vi "toml_to_value.vi"(8 "error in (no error)":errorcluster, 11 "toml line":string) -> (0 "error out":errorcluster, 1 "remaining":string, 2 "arg":string, 3 "token":T1)   [LabVIEW 2017]
uses:
  toml_token.ctl
  <vilib>/regexp/Match Regular Expression.xnode
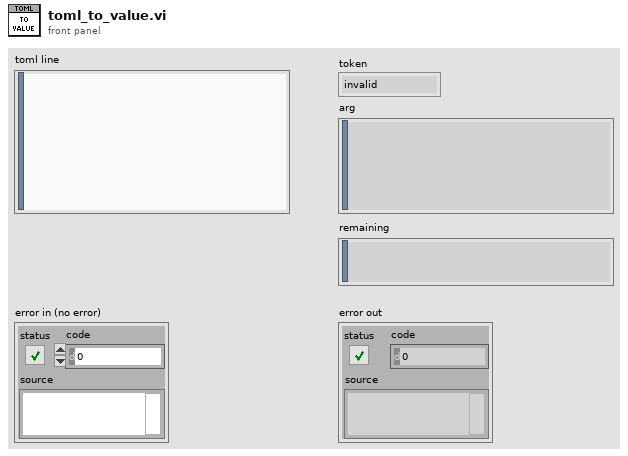
[diagram p1: front panel]
types:
  T1 = typedef "toml_token.ctl" = enum8{"invalid", "bool", "string", "string_start", "int", "uint", "float", "datetime", "array", "inline_table", "table", "table_element", "key", "comment", "comment_inline", "end"}
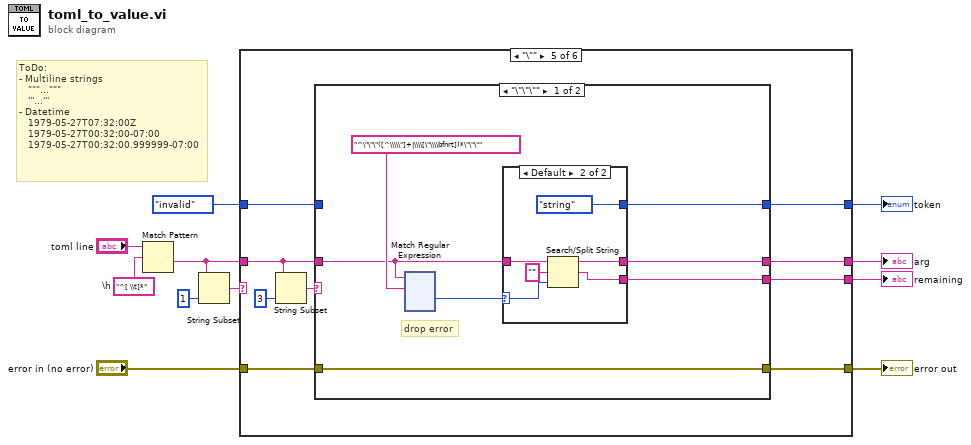
[diagram p0: block diagram]
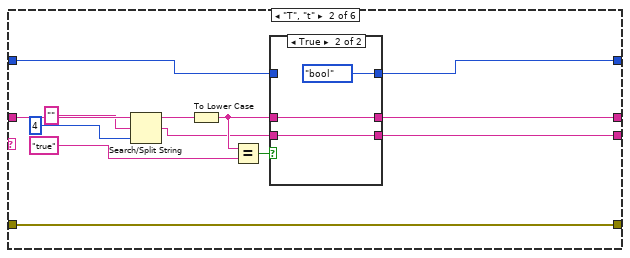
[diagram p3: hidden frame]
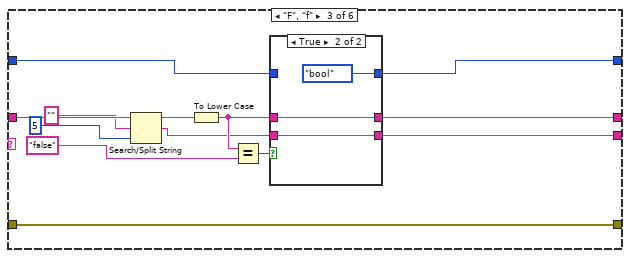
[diagram p5: hidden frame]
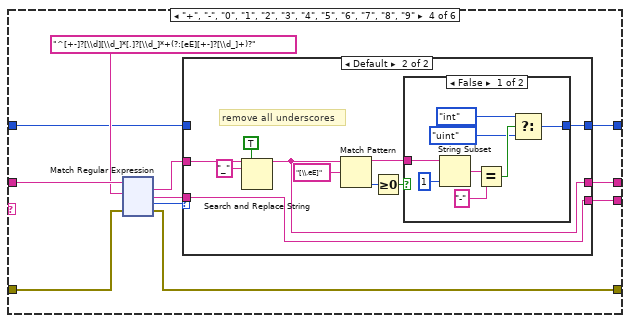
[diagram p7: hidden frame]
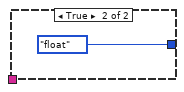
[diagram p9: hidden frame]
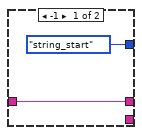
[diagram p10: hidden frame]
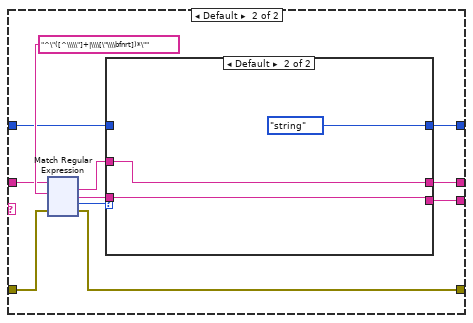
[diagram p11: hidden frame]
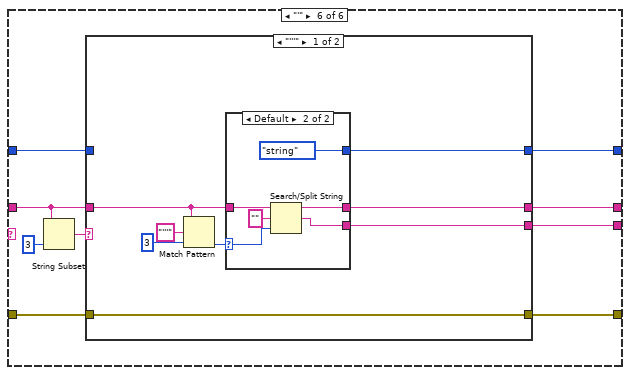
[diagram p13: hidden frame]
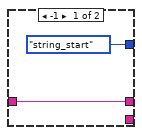
[diagram p14: hidden frame]
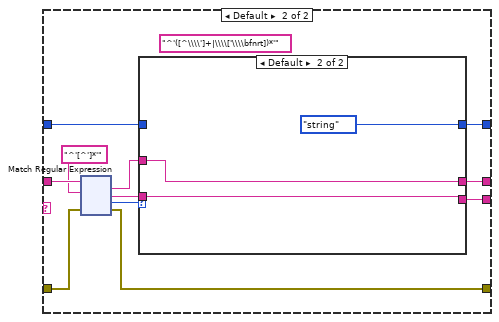
[diagram p15: hidden frame]
diagram:
  w11 = "^[ \\t]*"  # \h
  # "ToDo:\n- Multiline strings \n   \"\"\"...\"\"\"\n   '''...'''\n- Datetime\n   1979-05-27T07:32:00Z\n   1979-05-27T00:32:00-07:00\n   1979-05-27T00:32:00.999999-07:00"
  n1 = Match Pattern(string="toml line", regular expression=w11) -> (after substring=w7:string)  [unwired: 1 in, 3 out]
  n2 = String Subset(string=w7, length (rest)=1 ("length (rest)")) -> (substring=w8:string)  [unwired: 1 in]
  n3 = case shown="\"\\\"\"" w8 {
    tunnel: w7 -> [_ w25 w42 w58 w194 w461]
    tunnel: [_ w18 w35 w50 w197 w464] -> w6
    tunnel: [_ w15 w32 w49 w196 w463] -> w5
    tunnel: [w13 w21 w38 w53 w199 w466] -> w4
    tunnel: toml_token."invalid" ("token") -> [w13 w14 w31 w52 w198 w465]
    tunnel: [w12 w20 w37 w55 w200 w467] -> w2
    tunnel: "error in (no error)" -> [w12 w20 w37 w56 w201 w468]
    frame Default {
    }
    frame "T", "t" {
      n4 = Search/Split String(string=w25, search string/char (-)="", offset (0)=4 ("length (rest)")) -> (substring before match=w22:string, match + rest of string=w16:string)  [unwired: 1 out]
      n5 = To Lower Case(string=w22) -> (all lower case string=w17:string)
      n6 = Equal?(x=w17, y="true") -> (x = y?=w19:bool)
      n7 = case shown="True" w19 {
        tunnel: [w27 toml_token."bool" ("token")] -> w21
        tunnel: [_ w29] -> w18
        tunnel: w17 -> [_ w29]
        tunnel: w16 -> [_ w28]
        tunnel: [_ w28] -> w15
        tunnel: w14 -> [w27 _]
        frame False {
        }
        frame True {
        }
      }
    }
    frame "F", "f" {
      n8 = Search/Split String(string=w42, search string/char (-)="", offset (0)=5 ("length (rest)")) -> (substring before match=w39:string, match + rest of string=w33:string)  [unwired: 1 out]
      n9 = To Lower Case(string=w39) -> (all lower case string=w34:string)
      n10 = Equal?(x=w34, y="false") -> (x = y?=w36:bool)
      n11 = case shown="True" w36 {
        tunnel: [w44 toml_token."bool" ("token")] -> w38
        tunnel: [_ w46] -> w35
        tunnel: w34 -> [_ w46]
        tunnel: w33 -> [_ w45]
        tunnel: [_ w45] -> w32
        tunnel: w31 -> [w44 _]
        frame False {
        }
        frame True {
        }
      }
    }
    frame "+", "-", "0", "1", "2", "3", "4", "5", "6", "7", "8", "9" {
      n12 = xnode "Match Regular Expression"("input string"=w58, "regular expression"="^[+-]?[\\d][\\d_]*[.]?[\\d_]*+(?:[eE][+-]?[\\d_]+)?", "error in"=w56) -> ("whole match"=w51:string, "after match"=w48:string, "offset past match"=w54:i32, "error out"=w55:errorcluster)  [unwired: 3 in, 1 out]
      n13 = case shown="Default" w54 {
        tunnel: [w59 w65] -> w53
        tunnel: w52 -> [w59 _]
        tunnel: w51 -> [_ w63]
        tunnel: [_ w62] -> w50
        tunnel: [_ w64] -> w49
        tunnel: w48 -> [_ w64]
        frame -1 {
        }
        frame Default {
          # "remove all underscores"
          n14 = Search and Replace String(replace all?=TRUE ("replace all? (F)"), input string=w63, search string="_") -> (result string=w62:string)  [unwired: 5 in, 3 out]
          n15 = Match Pattern(string=w62, regular expression="[\\.eE]") -> (before substring=w66:string, offset past match=w68:i32)  [unwired: 1 in, 2 out]
          n16 = Greater Or Equal To 0?(x=w68) -> (x >= 0?=w67:bool)
          n17 = case shown="False" w67 {
            tunnel: w66 -> [w77 _]
            tunnel: [w72 toml_token."float" ("token")] -> w65
            frame False {
              n18 = String Subset(string=w77, length (rest)=1 ("length (rest)")) -> (substring=w75:string)  [unwired: 1 in]
              n19 = Equal?(x=w75, y="-") -> (x = y?=w73:bool)
              n20 = Select(t=toml_token."int" ("token"), s=w73, f=toml_token."uint" ("token")) -> (s? t:f=w72:T1)
            }
            frame True {
            }
          }
        }
      }
    }
    frame "\"" {
      n21 = String Subset(string=w194, length (rest)=3 ("length (rest)")) -> (substring=w193:string)  [unwired: 1 in]
      n22 = case shown="\"\\\"\\\"\\\"\"" w193 {
        tunnel: w201 -> [w208 w340]
        tunnel: [w208 w339] -> w200
        tunnel: [w207 w337] -> w199
        tunnel: w198 -> [_ w336]
        tunnel: [w206 w334] -> w197
        tunnel: [w205 w333] -> w196
        tunnel: w194 -> [w202 w331]
        frame "\"\"\"" {
          # "drop error"
          n23 = xnode "Match Regular Expression"("input string"=w202, "regular expression"="^\"\"\"([^\\\\\"]+|\\\\[\"\\\\bfnrt])*\"\"\"") -> ("offset past match"=w203:i32)  [unwired: 4 in, 4 out]
          n24 = case shown="Default" w203 {
            selector: w203 -> [_ w329]
            tunnel: w202 -> [w324 w330]
            tunnel: [w324 w327] -> w206
            tunnel: [_ w326] -> w205
            tunnel: [toml_token."string_start" ("token") toml_token."string" ("token")] -> w207
            frame -1 {
            }
            frame Default {
              n25 = Search/Split String(string=w330, search string/char (-)="", offset (0)=w329) -> (substring before match=w327:string, match + rest of string=w326:string)  [unwired: 1 out]
            }
          }
        }
        frame Default {
          n26 = xnode "Match Regular Expression"("input string"=w331, "regular expression"="^\"([^\\\\\"]+|\\\\[\"\\\\bfnrt])*\"", "error in"=w340) -> ("whole match"=w335:string, "after match"=w332:string, "offset past match"=w338:i32, "error out"=w339:errorcluster)  [unwired: 3 in, 1 out]
          n27 = case shown="Default" w338 {
            tunnel: [w342 toml_token."string" ("token")] -> w337
            tunnel: w336 -> [w342 _]
            tunnel: w335 -> [_ w344]
            tunnel: [_ w344] -> w334
            tunnel: [_ w343] -> w333
            tunnel: w332 -> [_ w343]
            frame -1 {
            }
            frame Default {
            }
          }
        }
      }
    }
    frame "'" {
      n28 = String Subset(string=w461, length (rest)=3 ("length (rest)")) -> (substring=w460:string)  [unwired: 1 in]
      n29 = case shown="\"'''\"" w460 {
        tunnel: w461 -> [w473 w495]
        tunnel: w468 -> [w476 w493]
        tunnel: [w476 w492] -> w467
        tunnel: [w469 w490] -> w466
        tunnel: w465 -> [_ w489]
        tunnel: [w471 w487] -> w464
        tunnel: [w470 w486] -> w463
        frame "'''" {
          n30 = Match Pattern(string=w473, regular expression="'''", offset (0)=3) -> (offset past match=w472:i32)  [unwired: 3 out]
          n31 = case shown="Default" w472 {
            selector: w472 -> [_ w483]
            tunnel: w473 -> [w478 w484]
            tunnel: [w478 w481] -> w471
            tunnel: [_ w480] -> w470
            tunnel: [toml_token."string_start" ("token") toml_token."string" ("token")] -> w469
            frame -1 {
            }
            frame Default {
              n32 = Search/Split String(string=w484, search string/char (-)="", offset (0)=w483) -> (substring before match=w481:string, match + rest of string=w480:string)  [unwired: 1 out]
            }
          }
        }
        frame Default {
          (unwired) "^'([^\\\\']+|\\\\['\\\\bfnrt])*'"
          n33 = xnode "Match Regular Expression"("input string"=w495, "regular expression"="^'[^']*'", "error in"=w493) -> ("whole match"=w488:string, "after match"=w485:string, "offset past match"=w491:i32, "error out"=w492:errorcluster)  [unwired: 3 in, 1 out]
          n34 = case shown="Default" w491 {
            tunnel: [w496 toml_token."string" ("token")] -> w490
            tunnel: w489 -> [w496 _]
            tunnel: w488 -> [_ w498]
            tunnel: [_ w498] -> w487
            tunnel: [_ w497] -> w486
            tunnel: w485 -> [_ w497]
            frame -1 {
            }
            frame Default {
            }
          }
        }
      }
    }
  }
  "error out" <- w2
  "token" <- w4
  "arg" <- w6
  "remaining" <- w5
